vi "Lookup Region.vi"() -> (3 "Region":T1)   [LabVIEW 2017]
uses:
  Regions Enum.ctl
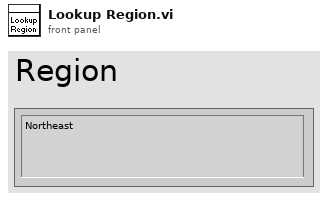
[diagram p1: front panel]
types:
  T1 = typedef "Regions Enum.ctl" = enum16{"Northeast", "Southeast", "North Central", "South Central", "Plains", "Northwest", "Southwest"}
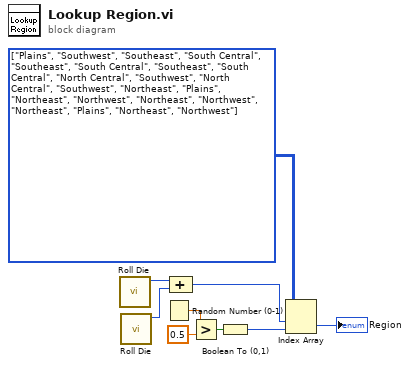
[diagram p0: block diagram]
diagram:
  w4 = T1[][] [[enum."Plains", enum."Southwest"], [enum."Southeast", enum."South Central"], [enum."Southeast", enum."South Central"], [enum."Southeast", enum."South Central"], [enum."North Central", enum."Southwest"], [enum."North Central", enum."Southwest"], [enum."Northeast", enum."Plains"], [enum."Northeast", enum."Northwest"], [enum."Northeast", enum."Northwest"], [enum."Northeast", enum."Plains"], [enum."Northeast", enum."Northwest"]] items=["Northeast", "Southeast", "North Central", "South Central", "Plains", "Northwest", "Southwest"]
  n1 = call "Roll Die.vi"() -> ("Number"=w5:i32)  [unwired: 11 in]
  n2 = call "Roll Die.vi"() -> ("Number"=w6:i32)  [unwired: 11 in]
  n3 = Random Number (0-1)() -> (number: 0 to 1=w7:dbl)
  n4 = Compound Arithmetic op=ADD(w5, w6) -> (w3:i32)
  n5 = Greater?(x=w7, y=0.5) -> (0:w9:bool)
  n6 = Boolean To (0,1)(Boolean=w9) -> (0, 1=w2:i16)
  n7 = Index Array(array=w4, index (row)=w3, index (col)=w2) -> (element=→"Region":T1)
